vi "Error.vi"(8 "error in (no error)":errorcluster, 11 "message queue in":T1) -> (0 "error out":errorcluster)   [LabVIEW 2015, in "Configuration Tool.lvlib"]
doc: "Enqueues the error as a message so it can be hanlde in the error caseCopyright 2017 National Instruments Corporation\n\nLicensed under the Apache License, Version 2.0 (the \"License\"); you may not use this file except in compliance with the License. You may obtain a copy of the License at http://www.apache.org/licenses/LICENSE-2.0\nUnless required by applicable law or agreed to in writing, software distributed under the License is distributed on an \"AS IS\" BASIS, WITHOUT WARRANTIES OR CONDITIONS OF ANY KIND, either express or implied. See the License for the specific language governing permissions and limitations under the License."
uses:
  Configuration Tool.lvlib
  <vilib>/NI/AMC/Message Queue.ctl
  <vilib>/NI/AMC/Message.ctl
  <vilib>/NI/Tools/Keyed Array/KeyedArray.ctl
  <vilib>/NI/AMC/Create Single Message.vi
  <vilib>/NI/AMC/Update Message Routing Info.vi
  <vilib>/NI/AMC/Send Message.vi
  <vilib>/NI/AMC/AMC.lvlib
  <vilib>/NI/Tools/Keyed Array/Tools_KeyedArray.lvlib
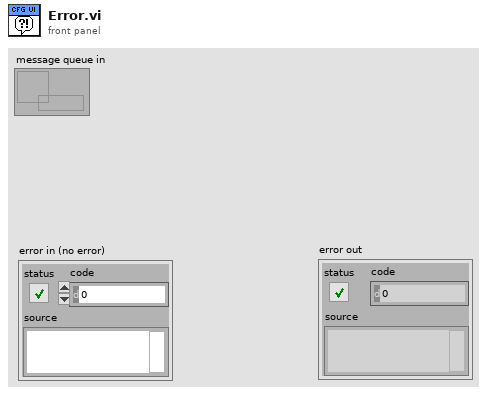
[diagram p1: front panel]
types:
  T1 = typedef "AMC.lvlib/Message Queue.ctl" = refnum<queue>
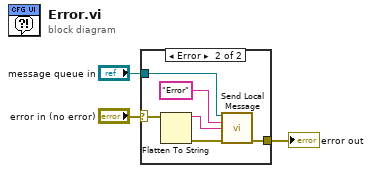
[diagram p0: block diagram]
diagram:
  n1 = case shown="Error" "error in (no error)" {
    selector: "error in (no error)" -> [_ w5]
    tunnel: [_ w9] -> w3
    tunnel: "message queue in" -> [_ w8]
    frame No Error {
    }
    frame Error {
      n2 = Flatten To String(anything=w5) -> (data string=w4:string, error out=w6:errorcluster)  [unwired: 3 in, 1 out]
      n3 = call <vilib>:"Send Local Message.vi"("message queue in"=w8, "message name"="Error", "message value"=w4, "error in"=w6) -> ("error out"=w9:errorcluster)  [unwired: 9 in, 2 out]
    }
  }
  "error out" <- w3
